vi "Exercise 6.3.vi"() -> ()   [LabVIEW 2010]
panel:
  out "Channel 2 Signal":dbl
  out "Channel 1 Signal":dbl
  in  "stop":bool
  in  "Filter 2":enum16{"Highpass", "Lowpass"}(ring)
  in  "Voltage 2":dbl(knob)=4.941296695804926 scale=0.0..10.0
  in  "Filter 1":enum16{"Highpass", "Lowpass"}(ring)=enum."Lowpass"
  in  "Voltage 1":dbl(knob)=4.803595814074423 scale=0.0..10.0
  in  "Filter 2":enum16{"Highpass", "Lowpass"}(ring)=enum."Lowpass"
  in  "Voltage 2":dbl(knob)=4.973040184713472 scale=0.0..10.0
  in  "Filter 1":enum16{"Highpass", "Lowpass"}(ring)=enum."Lowpass"
  in  "Voltage 1":dbl(knob)=5.047829554468576 scale=0.0..10.0
  # "Channel 1 Control"
  # "Channel 2 Control"
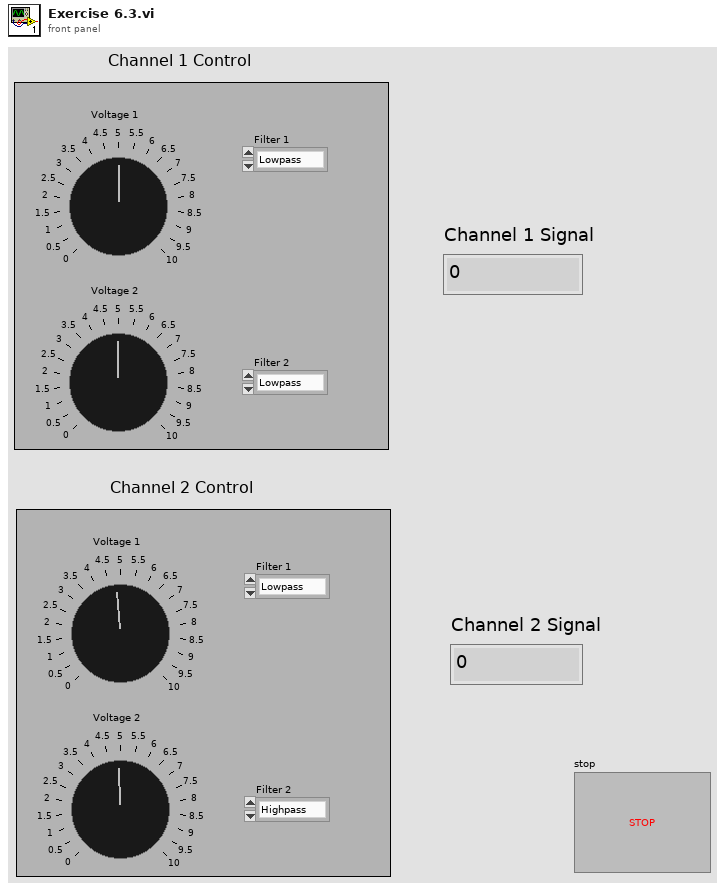
[diagram p1: front panel]
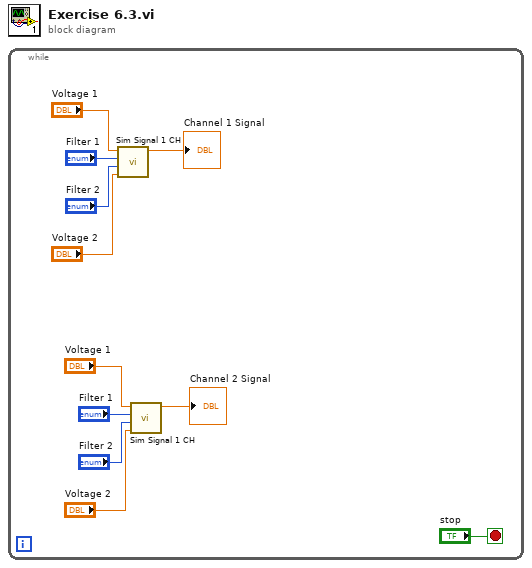
[diagram p0: block diagram]
diagram:
  n1 = while {
    stop <- "stop" stop-if-true
    n2 = call "Sim Signal 1 CH.vi"("Voltage 2"="Voltage 2", "Filter 2"="Filter 2", "Filter 1"="Filter 1", "Voltage 1"="Voltage 1") -> ("Signal 1 Out"=→"Channel 1 Signal":dbl)  [unwired: 7 in]
    n3 = call "Sim Signal 1 CH.vi"("Voltage 2"="Voltage 2", "Filter 2"="Filter 2", "Filter 1"="Filter 1", "Voltage 1"="Voltage 1") -> ("Signal 1 Out"=→"Channel 2 Signal":dbl)  [unwired: 7 in]
  }
